vi "def.hReadChannels-UandP-2013.vi"(0 "FPGA VI Reference In":refnum<k20>, 1 "SavGol side points":i32=10, 3 "Use Voltage or Power for AO?":bool, 4 "order polynomial":i32=2, 5 "Nsamples":u32=10000, 6 "error in":errorcluster, 8 "output cluster":T3, 9 "No. Of Samples to average":i32=10, 10 "variables cluster":T2, 11 "calculation settings":i32(slide) scale=0.0..3.0) -> (2 "Fehler":bool, 13 "AdjustedArray":sgl[][](array[numeric]), 18 "single channel voltage array":dbl[](array[numeric]), 19 "real time P_rad array":dbl[](array[numeric]), 20 "FPGA VI Reference Out":refnum<k20>, 22 "PowerArray":sgl[][](array[numeric]), 25 "RawArray":sgl[][](array[numeric]), 26 "error out":errorcluster)   [LabVIEW 2014]
doc: "startet das einlesen und führt dies bis n Samples aus\nHier mit FIFO und IRQ."
uses:
  <vilib>/Utility/error.llb/Error Cluster From Error Code.vi
  <vilib>/rvi/errors/niLvFpgaAdjustHostInterfaceError.vi
  <vilib>/RVI Host/nirviSupport.llb/nirviErrorClusterFromErrorCode.vi
  <vilib>/rvi/interface/nirviReadWriteControl/nirviReadWriteControl.xnode
  FPGA Bitfiles/W7XBolo2017_FPGATarget_fmain2014_DACRangeVoltage.lvbitx
  f_main_2014.vi
  <vilib>/rvi/interface/nirviMethod/nirviMethod.xnode
  NiFpgaLv.dll
  <vilib>/rvi/interface/nirviMethod/StockFPGA_InlinedMethodWaitForMultipleIRQ.vi
  <vilib>/FPGAPlugInAG/PCI-7813R/niLvFpga_WaitOnIrq_PCI-7813R.vi
  <vilib>/FPGAPlugInAG/PCI-7813R/niLvFpga_AcknowledgeIrq_PCI-7813R.vi
  <vilib>/FPGAPlugInAG/PCI-7813R/niLvFpga_ReadFifo_PCI-7813R.vi
  <vilib>/rvi/errors/niLvFpgaMergeErrorWithErrorCode.vi
panel:
  out "current P_rad [MW]":dbl
  out "current power":dbl[](array[numeric])
  out "single channel voltage * factor":dbl
  out "single channel voltage":dbl
  out "dU/dt":sgl[](array[numeric])
  out "channel number":i64
  in  "Tab Control":T1(tab)
  out "16bit integer voltage sample":i16[](array[numeric])=[-3459, -13133, -14604, -16468, 467, -1949, 12299, 12787, 12472, -19409, -24159, 19527, -14453, 13215, 13480, -17931, -19879, 19455, -20502, -24677, -3, 20022, 11523, 10117, 14450, -11995, -12638, 11593, -19028, 12318, 19839, -23479, 32767, -21197, -15773, 20123, 21626, -27672, 23062, -27030, 4395, 3490, 7778, -9544, 25980, -26635, -25599, 29504, 12544, -15434, 16294, -20022, -6530, 14029, -13674, -17269, -19063, -18202, -13922, 21944, -6026, -8393, -17071, -20550, 12209, -14874, -15412, 11029, -20655, 14995, 22414, -12873, 5782, -26944, -17259, 19698, -13837, 22149, 14480, -14147, -12057, 17536, 17816, -16154, -28940, -27971, -27523, -32768, -7372, 9053, 14111, -11921, 20354, -19665, -19289, 15438, -21905, 20094, 19557, -3, 18164, -14518, -19835, 24079, 10990, -13629, -14209, 12810, 4988, -72, 5308, -15, -12833, -7, -34, -7, -7, -11, -62, -4, -6, -7, -47, -5, -8, -29, -17, -1]
  out "RTPRad voltage factor":dbl
  out "Timed Out":bool
  out "STOP?":bool
  out "Elements Remaining":u32
  out "empty sample array":dbl[](array[numeric])
  out "Nsamples array":i64[](array[numeric])
  out "sample":i32
  out "new level of override":i32
  out "last U sample":sgl[](array[numeric])
  out "rt prad average array":dbl[][](array[numeric])
  out "element of channel\nand sample":sgl
  in  "magic number":dbl=1.0
  out "prad av array":dbl[](array[numeric])
  out "RawScal":dbl[](array[numeric])
  out "Scale(mV)":sgl[](array[numeric])
  out "SumScal":dbl[](array[numeric])
  out "Tau/dt":dbl[](array[numeric])
  out "F_ch":dbl[](array[numeric])
  out "tau_fact":dbl[](array[numeric])
  out "kbolott_and_volume":dbl[][](array[numeric])
  out "samples to exclude":u32
  out "single channel number":i64
  out "channelNumber":i32
  out "channelSelection":i64[][](array[numeric])
  out "tau_M":dbl[](array[numeric])
  out "Offsets":dbl[](array[numeric])
  out "SampleTime":sgl
  out "voltage factor":dbl
  out "Scale(mV) transf.":sgl[](array[numeric])
  out "V_cam":dbl
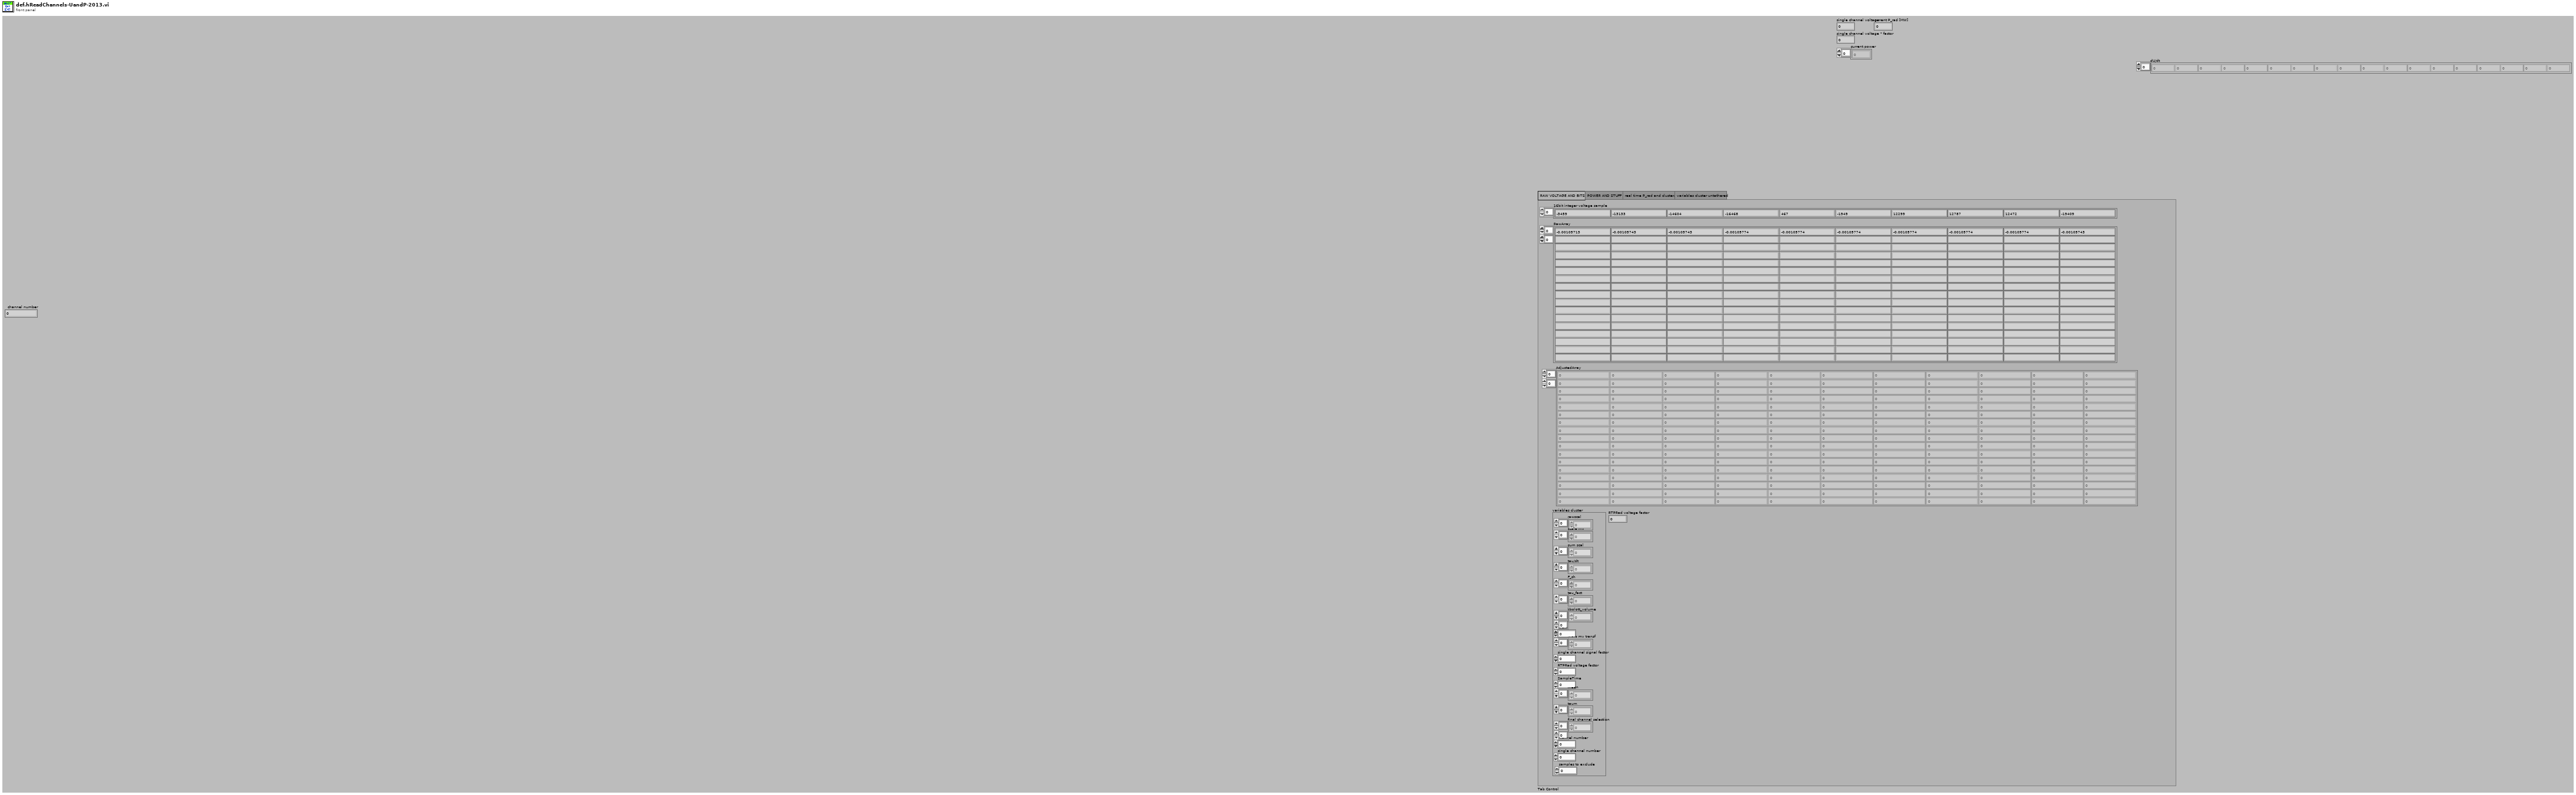
[diagram p1: front panel]
types:
  T1 = enum32{"RAW VOLTAGE AND BITS", "POWER AND STUFF", "real time P_rad and clusters", "variables cluster untathered"}
  T2 = cluster{"rawscal":dbl[], "scale mv":sgl[], "sum scal":dbl[], "tau/dt":dbl[], "F_ch":dbl[], "tau_fact":dbl[], "kbolott_volume":dbl[][], "Vcam":dbl, "scale mv transf":sgl[], "single channel signal factor":dbl, "RTPRad voltage factor":dbl, "SampleTime":sgl, "mean":dbl[], "taum":dbl[], "final channel selection":i64[][], "channel number":i32, "single channel number":i64, "samples to exclude":u32}
  T3 = cluster{"real time P_rad":refnum<vi>, "real time P_rad array":refnum<vi>, "single channel voltage":refnum<vi>, "single channel voltage array":refnum<vi>}
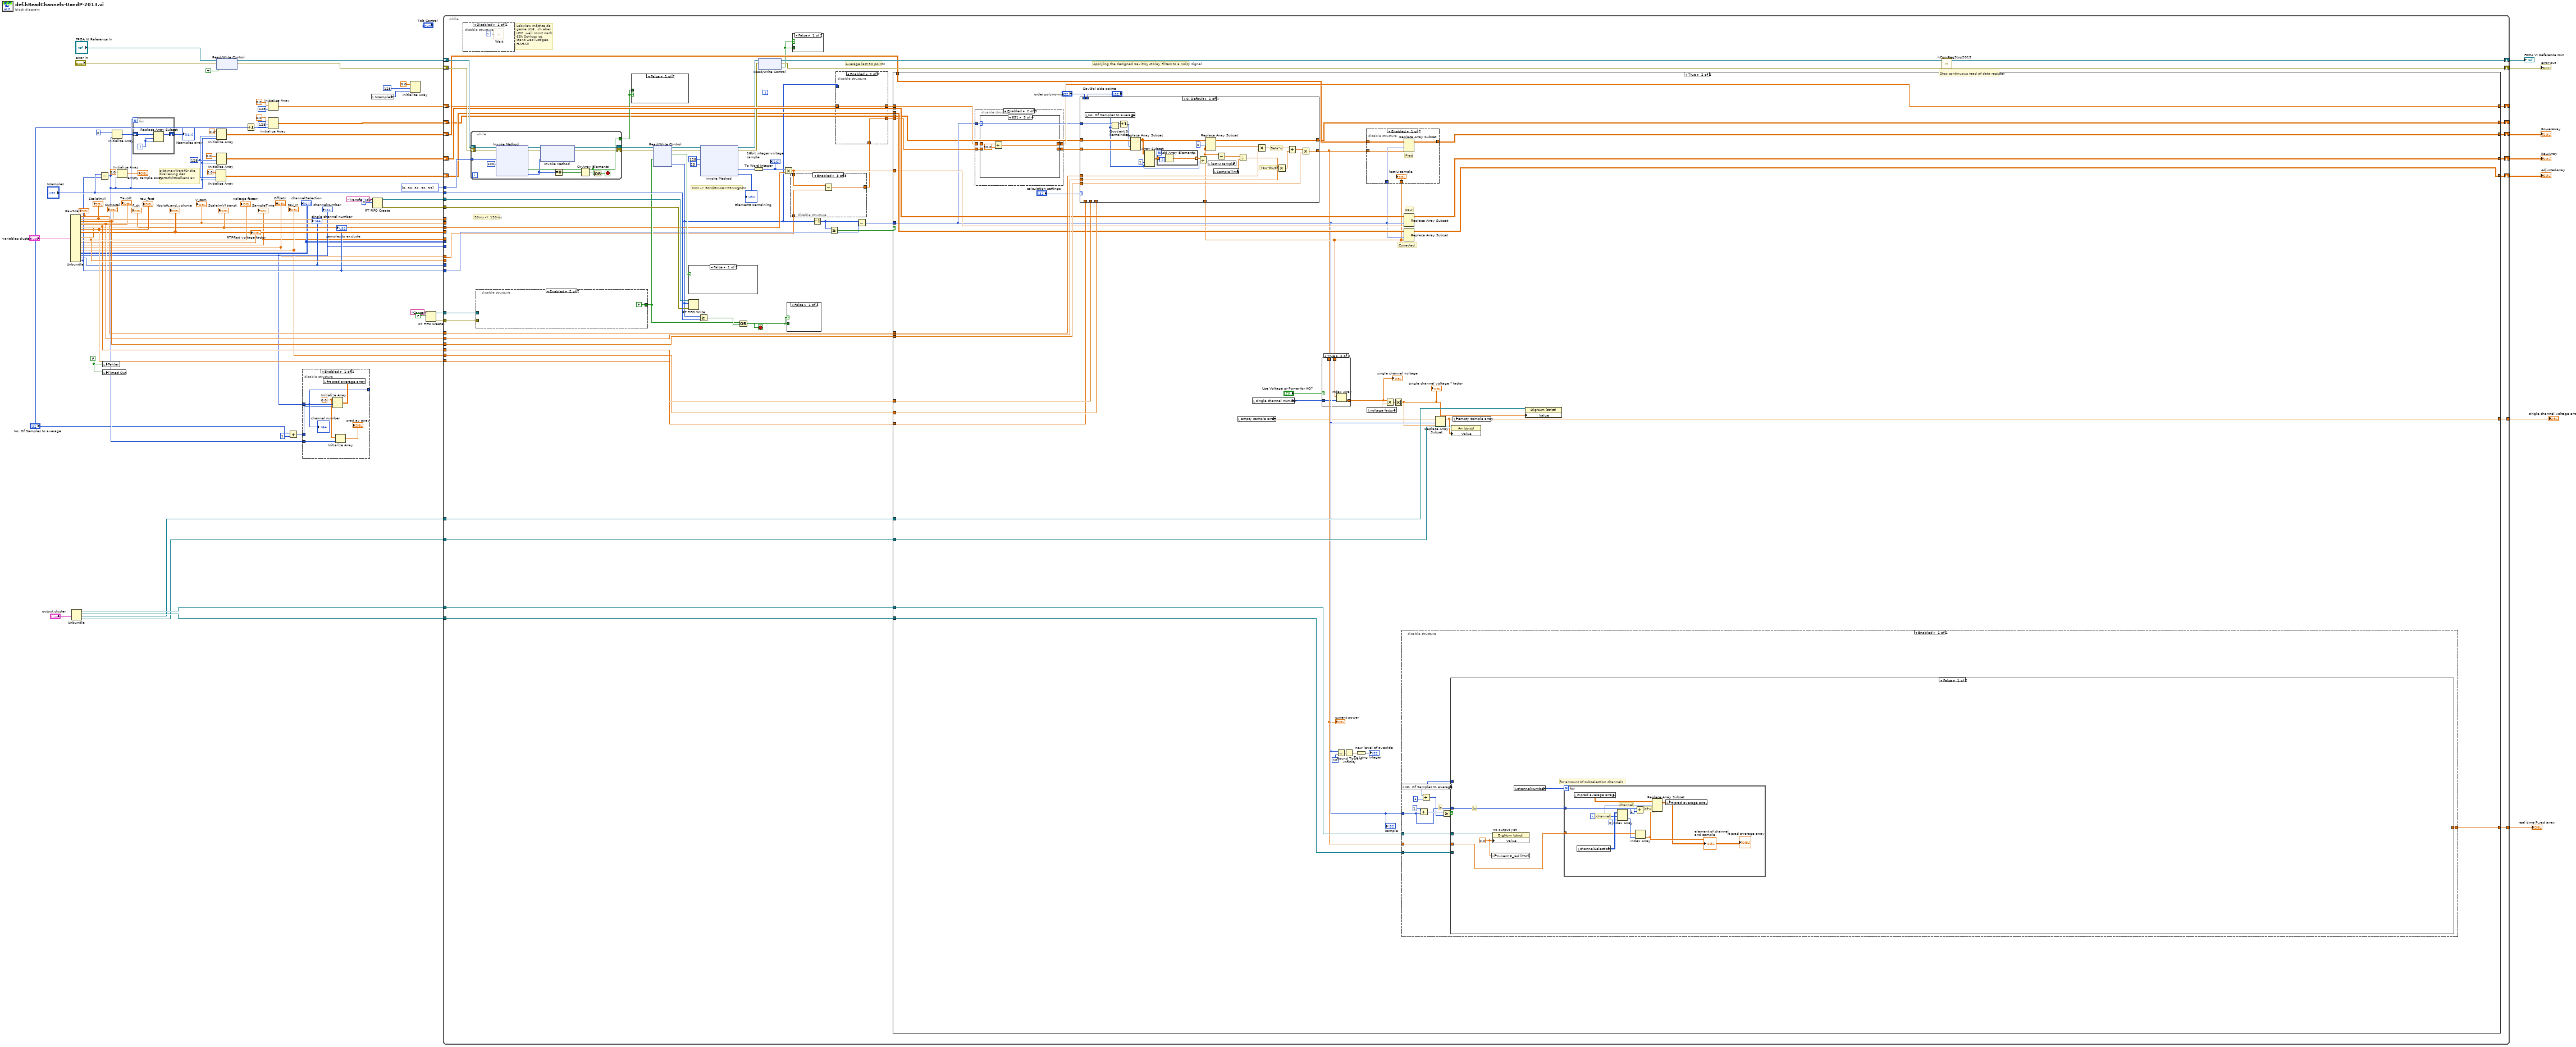
[diagram p0: block diagram]
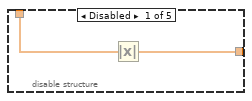
[diagram p2: hidden frame]
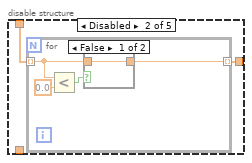
[diagram p3: hidden frame]
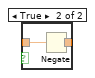
[diagram p4: hidden frame]
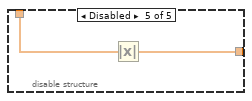
[diagram p6: hidden frame]
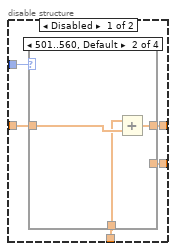
[diagram p7: hidden frame]
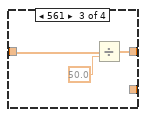
[diagram p9: hidden frame]
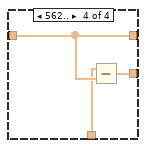
[diagram p10: hidden frame]
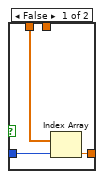
[diagram p12: hidden frame]
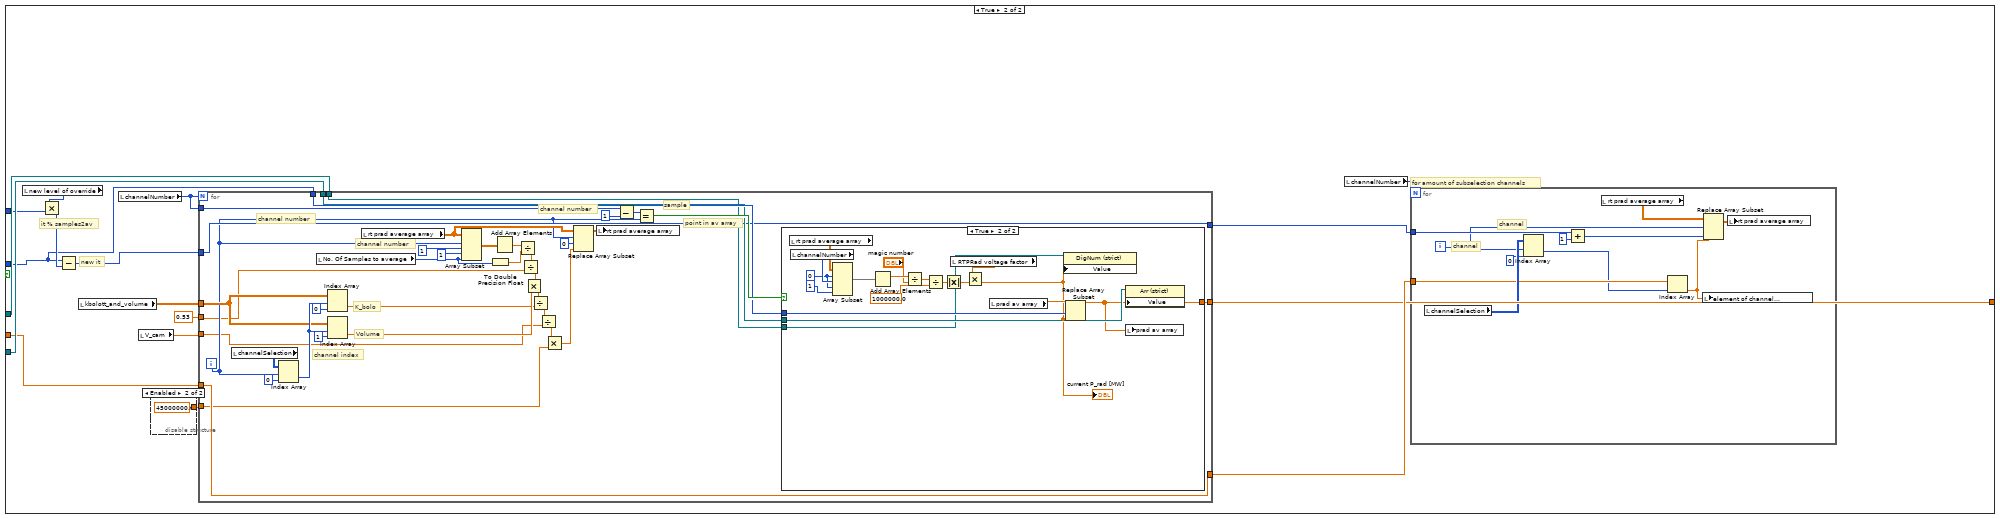
[diagram p13: hidden frame]
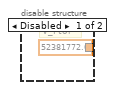
[diagram p14: hidden frame]
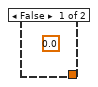
[diagram p15: hidden frame]
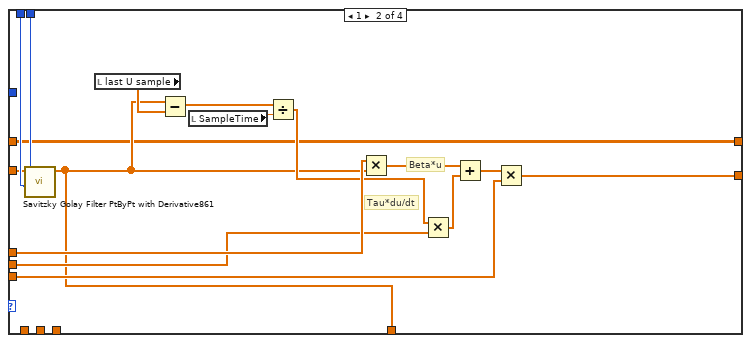
[diagram p17: hidden frame]
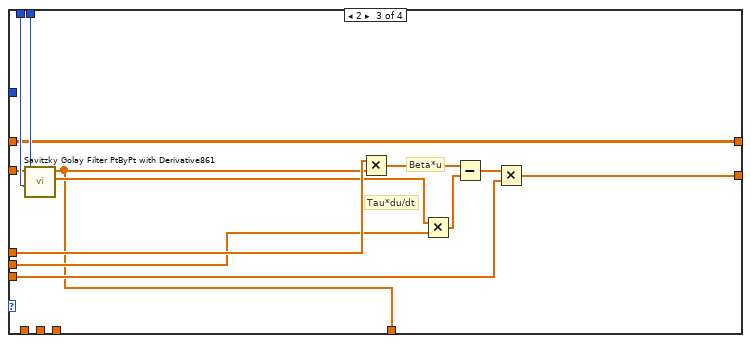
[diagram p18: hidden frame]
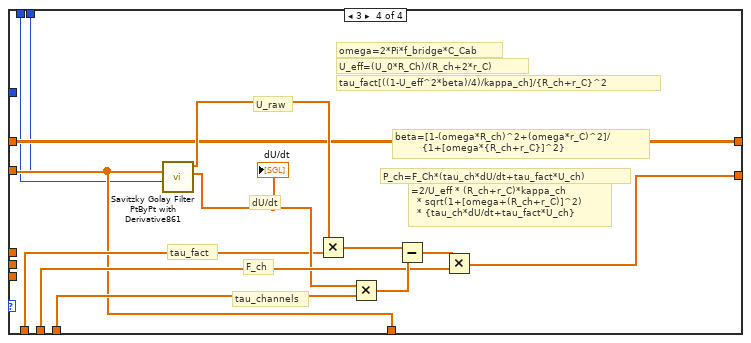
[diagram p19: hidden frame]
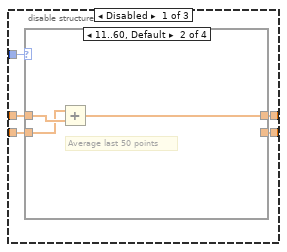
[diagram p20: hidden frame]
diagram:
  w44 = FALSE
  w19 = 128 ("dimension size")
  # "Stop continuous read of data register"
  # "gibt maxWert für die Skalierung des Fortschrittbalkens an"
  n1 = Unbundle("variables cluster") -> ("rawscal"=w35:dbl[], "scale mv"=w30:sgl[], "sum scal"=w36:dbl[], "tau/dt"=w34:dbl[], "F_ch"=w33:dbl[], "tau_fact"=w32:dbl[], "kbolott_volume"=w31:dbl[][], "Vcam"=w28:dbl, "scale mv transf"=w29:sgl[], "single channel signal factor"=w37:dbl, "RTPRad voltage factor"=→"RTPRad voltage factor":dbl, "SampleTime"=w8:sgl, "mean"=w9:dbl[], "taum"=w10:dbl[], "final channel selection"=w11:i64[][], "channel number"=w12:i32, "single channel number"=w13:i64, "samples to exclude"=w14:u32)
  "RawScal" <- w35
  "Scale(mV)" <- w30
  "SumScal" <- w36
  "Tau/dt" <- w34
  "F_ch" <- w33
  "tau_fact" <- w32
  "kbolott_and_volume" <- w31
  "V_cam" <- w28
  "Scale(mV) transf." <- w29
  "voltage factor" <- w37
  "SampleTime" <- w8
  "Offsets" <- w9
  "tau_M" <- w10
  "channelSelection" <- w11
  "channelNumber" <- w12
  "single channel number" <- w13
  "samples to exclude" <- w14
  n2 = Unbundle("output cluster") -> ("real time P_rad"=w39:refnum<vi>, "real time P_rad array"=w38:refnum<vi>, "single channel voltage"=w24:refnum<vi>, "single channel voltage array"=w23:refnum<vi>)
  n3 = Subtract(x="Nsamples", y=w14) -> (x-y=w18:u32)
  n4 = local write "Fehler"(w44) -> ()
  n5 = local write "Timed Out"(w44) -> ()
  n6 = Initialize Array(i64 0 ("element"), w18) -> (w46:i64[])
  n7 = Initialize Array(0.0 ("element"), w18) -> (→"empty sample array":dbl[])
  n8 = for {
    N: w18 -> [_]
    shift-right: [w76] -> w45
    shift-left: w46 -> [w78]
    i -> [w77]
    n9 = Replace Array Subset(array=w78, new element=w77, index=w77) -> (w76:i64[])
  }
  "Nsamples array" <- w45
  n10 = Initialize Array(sgl 0.0 ("element"), w19, w18) -> (w17:sgl[][])
  n11 = xnode "Read/Write Control"("FPGA VI Reference In"="FPGA VI Reference In", "error in"="error in", "ADCRead"=TRUE) -> ("FPGA VI Reference Out"=w57:refnum<k20>, "error out"=w56:errorcluster)
  n12 = Initialize Array(sgl 0.0 ("i"), w19, w18) -> (w66:sgl[][])
  n13 = Initialize Array(sgl 0.0, w19, w18) -> (w75:sgl[][])
  n14 = Increment(x="No. Of Samples to average") -> (x+1=w1:i32)
  n15 = Initialize Array(sgl 0.0 ("element"), 128 ("dimension size")) -> (w52:sgl[])
  n16 = Initialize Array(sgl 0.0 ("element"), 128 ("dimension size"), w1) -> (w3:sgl[][])
  n17 = Add(x="No. Of Samples to average", y=1) -> (x+y=w26:i32)
  n18 = disable-structure shown="Enabled" {
    disable-tunnel: w12 -> [w83]
    disable-tunnel: [w83] -> _
    disable-tunnel: w26 -> [w79]
    disable-tunnel: w18 -> [w80]
    frame Enabled {
      w82 = 0.0 ("element")
      n19 = Initialize Array(w82, w83, w79) -> (w84:dbl[][])
      n20 = local write "rt prad average array"(w84) -> ()
      n21 = Initialize Array(w82, w80) -> (→"prad av array":dbl[])
      "channel number" <- w83
    }
  }
  n22 = local read "Nsamples"() -> (w41:u32)
  n23 = RT FIFO Create(0:"Transferred1" ("name (unnamed)"), 1:u32 0) -> (8:w72:refnum<k33>, 11:w71:errorcluster)  [unwired: 2 in, 5 out]
  n24 = Initialize Array(sgl 0.0 ("element"), 128 ("dimension size"), w41) -> ()  [unwired: 1 out]
  n25 = RT FIFO Create(0:"Cancel" ("name (unnamed)"), 1:FALSE) -> (8:w69:refnum<k33>, 11:w68:errorcluster)  [unwired: 2 in, 5 out]
  n26 = while {
    tunnel: "Nsamples" -> [w139]
    shift-right: [w108] -> w15
    shift-left: w75 -> [w128]
    shift-right: [w140] -> w65
    shift-left: w57 -> [w143]
    shift-right: [w141] -> w64
    shift-left: w56 -> [w142]
    tunnel: w72 -> [w138]
    tunnel: w71 -> [w137]
    tunnel: w69 -> [w135]
    tunnel: w68 -> [w134]
    shift-right: [w132] -> w60
    shift-left: w66 -> [w133]
    tunnel: w29 -> [w127]
    tunnel: w34 -> [w87]
    tunnel: w36 -> [w126]
    tunnel: w35 -> [w125]
    shift-right: [w118] -> _
    shift-left: w52 -> [w94]
    tunnel: i32[] [0, 30, 31, 32, 33] -> [w113]
    tunnel: w23 -> [w110]
    tunnel: w24 -> [w109]
    tunnel: w13 -> [_]
    tunnel: w37 -> [_]
    tunnel: w9 -> [w88]
    tunnel: w14 -> [w89]
    tunnel: w39 -> [w105]
    tunnel: w38 -> [w100]
    tunnel: w33 -> [w104]
    tunnel: w32 -> [w103]
    tunnel: w30 -> [_]
    tunnel: w31 -> [_]
    tunnel: w8 -> [_]
    tunnel: w10 -> [w102]
    tunnel: w11 -> [_]
    tunnel: w12 -> [_]
    tunnel: w28 -> [_]
    tunnel: [w99] -> w22
    tunnel: [w98] -> w21
    shift-right: [w96] -> w16
    shift-left: w17 -> [w97]
    shift-right: [w85] -> _
    shift-left: w3 -> [w86]
    stop <- w114 stop-if-true
    # "Average last 50 points"
    # "Applying the designed Savitzky-Golay Filters to a noisy signal"
    # "LabView möchte da gerne U16, ich aber U32, weil sonst nach 65k Schluss ist. \nGanz was lustiges, HAHA!!"
    # "5ms=>25ms@MM"
    # "0ms -> 50ms"
    # "50ms -> 150ms"
    n27 = disable-structure shown="Disabled" {
      frame Disabled {
        n28 = call "Wait"("Count(uSec)"=u32 5) -> ()  [unwired: 1 out]
      }
      frame Enabled {
      }
    }
    n29 = while {
      tunnel: [w464] -> w117
      shift-right: [w466] -> w111
      shift-left: w143 -> [w473]
      shift-right: [w465] -> w112
      shift-left: w142 -> [w472]
      tunnel: w113 -> [w470]
      stop <- w463 stop-if-true
      n30 = xnode "Invoke Method"("FPGA VI Reference In"=w473, "error in"=w472, "IRQ Number(s)"=w470, "Timeout (ms)"=100) -> ("FPGA VI Reference Out"=w467:refnum<k20>, "error out"=w468:errorcluster, "Timed Out"=w464:bool, "IRQ(s) Asserted"=w469:i32[])
      n31 = xnode "Invoke Method"("FPGA VI Reference In"=w467, "error in"=w468, "IRQ Number(s)"=w469) -> ("FPGA VI Reference Out"=w466:refnum<k20>, "error out"=w465:errorcluster)
      n32 = Equal To 0?(x=w469) -> (x = 0?=w462:bool[])
      n33 = Or Array Elements(Boolean array=w462) -> (logical OR=w461:bool)
      n34 = Or(x=w461, y=w464) -> (x .or. y?=w463:bool)
    }
    n35 = disable-structure shown="Enabled" {
      disable-tunnel: [w479 FALSE] -> w136
      disable-tunnel: w135 -> [w478 _]
      disable-tunnel: w134 -> [w477 _]
      frame Disabled {
        # "Da es passieren kann, dass der letzte IRQ verschluckt wird, sichert dies der Timeoutwert von 50ms ab."
        n36 = RT FIFO Read(0:w478, 1:FALSE ("element"), 3:w477) -> (9:w479:bool)  [unwired: 5 out]
      }
      frame Enabled {
      }
    }
    n37 = case shown="False" w117 {
      tunnel: w117 -> [_ w481]
      frame False {
      }
      frame True {
        "Timed Out" <- w481
      }
    }
    n38 = xnode "Read/Write Control"("FPGA VI Reference In"=w111, "error in"=w112, "cancel"=w136) -> ("FPGA VI Reference Out"=w130:refnum<k20>, "error out"=w129:errorcluster, "Timeout"=w131:bool, "ScanID"=w95:u32)
    n39 = case shown="False" w131 {
      selector: w131 -> [_ w483]
      frame False {
      }
      frame True {
        n40 = local write "Fehler"(w483) -> ()
      }
    }
    n41 = RT FIFO Write(0:w138, 1:w95, 3:w137) -> ()  [unwired: 1 in, 5 out]
    n42 = Greater Or Equal?(x=w95, y=w139) -> (x >= y?=w144:bool)
    n43 = xnode ("Invoke Method")("FPGA VI Reference In"=w130, "error in"=w129, "Number of Elements"=u32 128, "Timeout (ms)"=25 ("Timeout")) -> ("FPGA VI Reference Out"=w120:refnum<k20>, "error out"=w119:errorcluster, "Data"=w122:u32[], "Elements Remaining"=→"Elements Remaining":u32)
    n44 = Compound Arithmetic op=OR(w136, w144) -> (w114:bool)
    n45 = To Word Integer(number=w122) -> (16bit integer=w121:i16[])
    "16bit integer voltage sample" <- w121
    n46 = xnode "Read/Write Control"("FPGA VI Reference In"=w120, "error in"=w119) -> ("FPGA VI Reference Out"=w140:refnum<k20>, "error out"=w141:errorcluster, "Fifo-Fehler"=w115:bool)
    n47 = Multiply(x=w121, y=w127) -> (x*y=w92:sgl[])
    n48 = case shown="False" w114 {
      tunnel: w114 -> [_ w474]
      frame False {
      }
      frame True {
        "STOP?" <- w474
      }
    }
    n49 = disable-structure shown="Enabled" {
      disable-tunnel: [w146 w147 w158 w159 w161] -> w91
      disable-tunnel: w92 -> [w145 w148 w157 w159 w160]
      disable-tunnel: w88 -> [_ _ w156 _ _]
      frame Disabled {
        n50 = Absolute Value(x=w145) -> (abs(x)=w146:sgl[])
      }
      frame Disabled {
        n51 = for {
          tunnel: w148 -> [w150] mode=indexing
          tunnel: [w149] -> w147 mode=indexing
          n52 = Less?(x=w150, y=sgl 0.0) -> (x < y?=w151:bool)
          n53 = case shown="False" w151 {
            tunnel: w150 -> [w153 w155]
            tunnel: [w153 w154] -> w149
            frame False {
            }
            frame True {
              n54 = Negate(x=w155) -> (-x=w154:sgl)
            }
          }
        }
      }
      frame Enabled {
        n55 = Subtract(x=w157, y=w156) -> (x-y=w158:dbl[])
      }
      frame Disabled {
      }
      frame Disabled {
        n56 = Absolute Value(x=w160) -> (abs(x)=w161:sgl[])
      }
    }
    n57 = case shown="False" w115 {
      tunnel: w115 -> [_ w475]
      frame False {
      }
      frame True {
        "Fehler" <- w475
      }
    }
    n58 = Decrement(x=w95) -> (x-1=w106:u32)
    n59 = Greater Or Equal?(x=w106, y=w89) -> (x >= y?=w107:bool)
    n60 = disable-structure shown="Enabled" {
      disable-tunnel: [w166 w178] -> w93
      disable-tunnel: w94 -> [w165 w178]
      disable-tunnel: w95 -> [w164 _]
      disable-tunnel: [w163 w177] -> w90
      disable-tunnel: w91 -> [w162 w177]
      frame Disabled {
        n61 = case shown="501..560, Default" w164 {
          tunnel: w162 -> [_ w168 _ w174]
          tunnel: [w167 w170 w171 w175] -> w166
          tunnel: w165 -> [w167 w169 w173 w175]
          tunnel: [_ _ _ w176] -> w163
          frame 0..500 {
          }
          frame 501..560, Default {
            n62 = Add(x=w168, y=w169) -> (x+y=w170:dbl[])
          }
          frame 561 {
            n63 = Divide(x=w173, y=sgl 50.0) -> (x/y=w171:dbl[])
          }
          frame 562.. {
            n64 = Subtract(x=w174, y=w175) -> (x-y=w176:dbl[])
          }
        }
      }
      frame Enabled {
      }
    }
    n65 = Subtract(x=w106, y=w89) -> (x-y=w101:u32)
    n66 = case shown="True" w107 {
      tunnel: w133 -> [w182 w218]
      tunnel: [w182 w219] -> w132
      tunnel: w128 -> [w181 w217]
      tunnel: w126 -> [_ w225]
      tunnel: w125 -> [_ w224]
      tunnel: w87 -> [_ w223]
      tunnel: [w183 w222] -> w118
      tunnel: w93 -> [w183 w206]
      tunnel: w92 -> [_ w205]
      tunnel: w110 -> [_ w221]
      tunnel: w109 -> [_ w220]
      tunnel: [w181 w216] -> w108
      tunnel: w101 -> [_ w203]
      tunnel: w105 -> [_ w212]
      tunnel: w100 -> [_ w211]
      tunnel: w104 -> [_ w215]
      tunnel: w103 -> [_ w213]
      tunnel: w102 -> [_ w214]
      tunnel: [_ w210] -> w99
      tunnel: [_ w209] -> w98
      tunnel: w97 -> [w180 w208]
      tunnel: [w180 w207] -> w96
      tunnel: w90 -> [_ w204]
      tunnel: w86 -> [w179 w202]
      tunnel: [w179 w201] -> w85
      frame False {
      }
      frame True {
        # "Corrected"
        # "Raw"
        n67 = disable-structure shown="Enabled" {
          disable-tunnel: [w416 w442 w453] -> w222
          disable-tunnel: w206 -> [w415 w441 w453]
          disable-tunnel: w203 -> [w414 w440 _]
          disable-tunnel: [w413 w439 w454] -> w196
          disable-tunnel: w204 -> [w412 w438 w454]
          frame Disabled {
            n68 = case shown="11..60, Default" w414 {
              tunnel: w412 -> [_ w418 _ w434]
              tunnel: [w417 w420 w422 w433] -> w416
              tunnel: w415 -> [w417 w419 w424 w433]
              tunnel: [_ _ _ w432] -> w413
              frame 0..10 {
              }
              frame 11..60, Default {
                # "Average last 50 points"
                n69 = Add(x=w418, y=w419) -> (x+y=w420:dbl[])
              }
              frame 61 {
                n70 = Divide(x=w424, y=sgl 50.0) -> (x/y=w421:dbl[])
                n71 = disable-structure shown="Enabled" {
                  disable-tunnel: [w425 w430] -> w422
                  disable-tunnel: w421 -> [w429 w430]
                  frame Disabled {
                    n72 = Initialize Array(2e-06 ("element"), 128 ("dimension size")) -> (w426:dbl[])
                    n73 = Subtract(x=w429, y=w426) -> (x-y=w425:dbl[])
                  }
                  frame Enabled {
                  }
                }
              }
              frame 62.. {
                n74 = Subtract(x=w434, y=w433) -> (x-y=w431:dbl[])
                n75 = disable-structure shown="Enabled" {
                  disable-tunnel: [w436 w437] -> w432
                  disable-tunnel: w431 -> [w435 w437]
                  frame Disabled {
                    n76 = Absolute Value(x=w435) -> (abs(x)=w436:dbl[])
                  }
                  frame Enabled {
                  }
                }
              }
            }
          }
          frame Enabled {
            n77 = case shown="651" w440 {
              tunnel: w438 -> [_ w444 _ w452]
              tunnel: [w443 w446 w447 w451] -> w442
              tunnel: w441 -> [w443 w445 w449 w451]
              tunnel: [_ _ _ w450] -> w439
              frame 0..600 {
              }
              frame 601..650, Default {
                # "Average last 50 points"
                n78 = Add(x=w444, y=w445) -> (x+y=w446:dbl[])
              }
              frame 651 {
                n79 = Divide(x=w449, y=sgl 50.0) -> (x/y=w447:dbl[])
              }
              frame 652.. {
                n80 = Subtract(x=w452, y=w451) -> (x-y=w450:dbl[])
              }
            }
          }
          frame Disabled {
          }
        }
        n81 = case shown="0, Default" "calculation settings" {
          tunnel: w225 -> [w367 w385 w398 _]
          tunnel: w224 -> [w366 w384 w397 _]
          tunnel: w223 -> [w365 w383 w396 _]
          tunnel: [w364 w382 w395 w403] -> w199
          tunnel: "SavGol side points" -> [_ w381 w394 w400]
          tunnel: "order polynomial" -> [_ w380 w393 w399]
          tunnel: w196 -> [w363 w379 w392 w401]
          tunnel: w203 -> [w362 _ _ _]
          tunnel: w202 -> [w361 w370 w387 w402]
          tunnel: [w360 w370 w387 w402] -> w201
          tunnel: [w359 w371 w386 w401] -> w200
          tunnel: w214 -> [_ _ _ w407]
          tunnel: w215 -> [_ _ _ w406]
          tunnel: w213 -> [_ _ _ w404]
          frame 0, Default {
            # "Beta*u"
            # "Tau*du/dt"
            n82 = local read "No. Of Samples to average"() -> (w353:i32)
            n83 = Quotient & Remainder(x=w362, y=w353) -> (x-y*floor(x/y)=w357:u32)  [unwired: 1 out]
            n84 = Increment(x=w357) -> (x+1=w358:u32)
            n85 = Replace Array Subset(array=w361, new element=w363, index (col)=w358) -> (w352:sgl[][])  [unwired: 1 in]
            n86 = Array Subset(array=w352, index (col)=1 ("index"), length (col)=w353) -> (w355:sgl[][])  [unwired: 2 in]
            n87 = for {
              tunnel: w355 -> [w369] mode=indexing
              tunnel: [w368] -> w354 mode=indexing
              n88 = Add Array Elements(numeric array=w369) -> (sum=w368:sgl)
            }
            n89 = Divide(x=w354, y=w353) -> (x/y=w359:sgl[])
            n90 = Replace Array Subset(array=w352, new element=w359, index (col)=0 ("index")) -> (w360:sgl[][])  [unwired: 1 in]
            n91 = local read "last U sample"() -> (w350:sgl[])
            n92 = local read "SampleTime"() -> (w348:sgl)
            n93 = Subtract(x=w359, y=w350) -> (x-y=w349:sgl[])
            n94 = Divide(x=w349, y=w348) -> (x/y=w344:sgl[])
            n95 = Multiply(x=w359, y=w366) -> (x*y=w347:dbl[])
            n96 = Multiply(x=w344, y=w365) -> (x*y=w345:dbl[])
            n97 = Add(x=w347, y=w345) -> (x+y=w346:dbl[])
            n98 = Multiply(x=w346, y=w367) -> (x*y=w364:dbl[])
          }
          frame 1 {
            # "Beta*u"
            # "Tau*du/dt"
            n99 = call "Savitzky Golay Filter PtByPt with Derivative861.vi"("order polynomial"=w380, "side points"=w381, "x"=w379) -> ("Filtered x"=w371:dbl[])  [unwired: 1 in, 7 out]
            n100 = local read "last U sample"() -> (w373:sgl[])
            n101 = Subtract(x=w371, y=w373) -> (x-y=w374:dbl[])
            n102 = local read "SampleTime"() -> (w372:sgl)
            n103 = Divide(x=w374, y=w372) -> (x/y=w376:dbl[])
            n104 = Multiply(x=w384, y=w371) -> (x*y=w378:dbl[])
            n105 = Multiply(x=w376, y=w383) -> (x*y=w375:dbl[])
            n106 = Add(x=w378, y=w375) -> (x+y=w377:dbl[])
            n107 = Multiply(x=w377, y=w385) -> (x*y=w382:dbl[])
          }
          frame 2 {
            # "Beta*u"
            # "Tau*du/dt"
            n108 = call "Savitzky Golay Filter PtByPt with Derivative861.vi"("order polynomial"=w393, "side points"=w394, "x"=w392) -> ("Filtered Derivative"=w388:dbl[], "Filtered x"=w386:dbl[])  [unwired: 1 in, 6 out]
            n109 = Multiply(x=w397, y=w386) -> (x*y=w391:dbl[])
            n110 = Multiply(x=w388, y=w396) -> (x*y=w389:dbl[])
            n111 = Subtract(x=w391, y=w389) -> (x-y=w390:dbl[])
            n112 = Multiply(x=w390, y=w398) -> (x*y=w395:dbl[])
          }
          frame 3 {
            # "beta=[1-(omega*R_ch)^2+(omega*r_C)^2]/\n         {1+[omega*{R_ch+r_C}]^2}"
            # "tau_fact[((1-U_eff^2*beta)/4)/kappa_ch]/{R_ch+r_C}^2"
            # "U_eff=(U_0*R_Ch)/(R_ch+2*r_C)"
            # "omega=2*Pi*f_bridge*C_Cab"
            # "=2/U_eff * (R_ch+r_C)*kappa_ch\n  * sqrt(1+[omega+(R_ch+r_C)]^2)\n  * {tau_ch*dU/dt+tau_fact*U_ch}"
            # "P_ch=F_Ch*(tau_ch*dU/dt+tau_fact*U_ch)"
            # "tau_channels"
            # "F_ch"
            # "tau_fact"
            # "U_raw"
            # "dU/dt"
            n113 = call "Savitzky Golay Filter PtByPt with Derivative861.vi"("order polynomial"=w399, "side points"=w400, "x"=w401) -> ("Filtered Derivative"=w405:dbl[], "Filtered x"=w408:dbl[])  [unwired: 1 in, 6 out]
            "dU/dt" <- w405
            n114 = Multiply(x=w408, y=w404) -> (x*y=w411:dbl[])
            n115 = Multiply(x=w405, y=w407) -> (x*y=w409:dbl[])
            n116 = Subtract(x=w411, y=w409) -> (x-y=w410:dbl[])
            n117 = Multiply(x=w410, y=w406) -> (x*y=w403:dbl[])
          }
        }
        "current power" <- w199
        n118 = local read "empty sample array"() -> (w192:dbl[])
        n119 = local read "single channel number"() -> (w194:i64)
        n120 = case shown="True" "Use Voltage or Power for AO?" {
          tunnel: w194 -> [w226 w231]
          tunnel: [w227 w230] -> w191
          tunnel: w200 -> [_ w229]
          tunnel: w199 -> [w228 _]
          frame False {
            n121 = Index Array(array=w228, index=w226) -> (element=w227:dbl)
          }
          frame True {
            n122 = Index Array(array=w229, index=w231) -> (element=w230:dbl)
          }
        }
        "single channel voltage" <- w191
        n123 = Divide(x=w203, y=10) -> (x/y=w187:dbl)
        n124 = Round Toward -Infinity(1:w187) -> (0:w188:dbl)
        n125 = To Long Integer(number=w188) -> (32bit integer=→"new level of override":i32)
        n126 = disable-structure shown="Enabled" {
          disable-tunnel: w218 -> [w459 w460]
          disable-tunnel: [w458 w460] -> w219
          disable-tunnel: w203 -> [w457 _]
          disable-tunnel: w199 -> [w456 _]
          disable-tunnel: w200 -> [w455 _]
          frame Enabled {
            # "Prad"
            n127 = Replace Array Subset(array=w459, new element=w456, index (col)=w457) -> (w458:sgl[][])  [unwired: 1 in]
            "last U sample" <- w455
          }
          frame Disabled {
          }
        }
        n128 = local read "voltage factor"() -> (w193:dbl)
        n129 = Multiply(x=w191, y=w193) -> (x*y=w190:dbl)
        n130 = Absolute Value(x=w190) -> (abs(x)=w184:dbl)
        "single channel voltage * factor" <- w184
        n131 = disable-structure shown="Enabled" {
          disable-tunnel: w203 -> [w236 _]
          disable-tunnel: w212 -> [w239 _]
          disable-tunnel: w211 -> [w238 _]
          disable-tunnel: w199 -> [w237 _]
          disable-tunnel: [w232 _] -> w210
          frame Enabled {
            # "it"
            n132 = local read "No. Of Samples to average"() -> (w233:i32)
            n133 = Add(x=1, y=w236) -> (x+y=w240:u32)
            n134 = Add(x=w233, y=i64 1) -> (x+y=w234:i64)
            n135 = Greater Or Equal?(x=w240, y=w234) -> (x >= y?=w242:bool)
            n136 = case shown="False" w242 {
              tunnel: w236 -> [w244 w261]
              tunnel: w239 -> [w246 w263]
              tunnel: w238 -> [_ w264]
              tunnel: w237 -> [w245 w262]
              tunnel: w233 -> [_ w260]
              tunnel: [_ w259] -> w232
              frame False {
                w243 = 0.0 ("Value")
                # "it"
                # "for amount of subselection channels"
                # "no output yet"
                n137 = local write "current P_rad [MW]"(w243) -> ()
                n138 = property class="DigNum (strict)"(reference=w246, "Value"=w243) -> ()  [unwired: 1 in, 2 out]
                n139 = local read "channelNumber"() -> (w247:i32)
                n140 = for {
                  N: w247 -> [_]
                  tunnel: w244 -> [w254]
                  tunnel: w245 -> [w252]
                  i -> [w249]
                  # "channel"
                  # "channel"
                  # "it+1"
                  n141 = local read "rt prad average array"() -> (w253:dbl[][])
                  n142 = local read "channelSelection"() -> (w258:i64[][])
                  n143 = Index Array(array=w258, index (row)=w249, index (col)=0 ("disabled index (col)")) -> (element=w248:i64)
                  n144 = Add(x=w254, y=1) -> (x+y=w255:u32)
                  n145 = Index Array(array=w252, index=w248) -> (element=w251:dbl)
                  "element of channel\nand sample" <- w251
                  n146 = Replace Array Subset(array=w253, new element=w251, index (row)=w249, index (col)=w255) -> (w250:dbl[][])
                  "rt prad average array" <- w250
                  n147 = local write "rt prad average array"(w250) -> ()
                }
              }
              frame True {
                # "new it"
                # "it % samples2av"
                # "for amount of subselection channels"
                n148 = local read "new level of override"() -> (w274:i32)
                n149 = Multiply(x=w274, y=w260) -> (x*y=w273:i32)
                n150 = Subtract(x=w261, y=w273) -> (x-y=w271:u32)
                n151 = local read "kbolott_and_volume"() -> (w272:dbl[][])
                n152 = local read "channelNumber"() -> (w266:i32)
                n153 = local read "V_cam"() -> (w268:dbl)
                n154 = disable-structure shown="Enabled" {
                  disable-tunnel: [52381772.0 45000000.0] -> w270
                  frame Disabled {
                    # "V_Ptor"
                  }
                  frame Enabled {
                  }
                }
                n155 = for {
                  N: w266 -> [_]
                  tunnel: w272 -> [w309]
                  tunnel: [w314] -> w267
                  tunnel: w262 -> [w314]
                  tunnel: [w294] -> w265
                  tunnel: w271 -> [w294]
                  tunnel: w270 -> [w288]
                  tunnel: 0.53 -> [w292]
                  tunnel: w268 -> [w289]
                  tunnel: w266 -> [w295]
                  tunnel: w261 -> [w300]
                  tunnel: w264 -> [w299]
                  tunnel: w263 -> [w296]
                  tunnel: [w279] -> w259
                  i -> [w293]
                  # "channel number"
                  # "channel number"
                  # "point in av array"
                  # "sample"
                  # "channel number"
                  # "K_bolo"
                  # "Volume"
                  # "channel index"
                  n156 = local read "channelSelection"() -> (w313:i64[][])
                  n157 = Index Array(array=w313, index (row)=w293, index (col)=0 ("disabled index (col)")) -> (element=w310:i64)
                  n158 = local read "No. Of Samples to average"() -> (w281:i32)
                  n159 = Index Array(array=w309, index (row)=w310, index (col)=0 ("disabled index (col)")) -> (element=w290:dbl)
                  n160 = Index Array(array=w309, index (row)=w310, index (col)=1 ("disabled index (col)")) -> (element=w291:dbl)
                  n161 = local read "rt prad average array"() -> (w304:dbl[][])
                  n162 = Array Subset(array=w304, index (row)=w293, length (row)=1, index (col)=1 ("index"), length (col)=w281) -> (w305:dbl[][])
                  n163 = To Double Precision Float(number=w281) -> (double precision float=w280:dbl)
                  n164 = Add Array Elements(numeric array=w305) -> (sum=w286:dbl)
                  n165 = Divide(x=w286, y=w280) -> (x/y=w278:dbl)
                  n166 = Divide(x=w278, y=w292) -> (x/y=w285:dbl)
                  n167 = Multiply(x=w285, y=w291) -> (x*y=w284:dbl)
                  n168 = Divide(x=w284, y=w290) -> (x/y=w283:dbl)
                  n169 = Divide(x=w283, y=w289) -> (x/y=w282:dbl)
                  n170 = Multiply(x=w282, y=w288) -> (x*y=w287:dbl)
                  n171 = Replace Array Subset(array=w304, new element=w287, index (row)=w293, index (col)=0 ("disabled index (col)")) -> (w302:dbl[][])
                  n172 = local write "rt prad average array"(w302) -> ()
                  n173 = Subtract(x=w295, y=i64 1) -> (x-y=w298:i64)
                  n174 = Equal?(x=w298, y=w293) -> (x = y?=w301:bool)
                  n175 = case shown="True" w301 {
                    tunnel: w300 -> [_ w329]
                    tunnel: w299 -> [_ w328]
                    tunnel: w296 -> [_ w327]
                    tunnel: [_ w318] -> w279
                    frame False {
                      (unwired) 0.0
                    }
                    frame True {
                      w324 = 0 ("index")
                      n176 = local read "rt prad average array"() -> (w330:dbl[][])
                      n177 = local read "channelNumber"() -> (w325:i32)
                      n178 = Array Subset(array=w330, index (row)=w324, length (row)=w325, index (col)=w324, length (col)=1 ("index")) -> (w332:dbl[][])
                      n179 = Add Array Elements(numeric array=w332) -> (sum=w322:dbl)
                      n180 = Divide(x=w322, y="magic number") -> (x/y=w323:dbl)
                      n181 = Divide(x=w323, y=1000000.0) -> (x/y=w319:dbl)
                      n182 = Absolute Value(x=w319) -> (abs(x)=w317:dbl)
                      n183 = local read "RTPRad voltage factor"() -> (w316:dbl)
                      n184 = Multiply(x=w316, y=w317) -> (x*y=w315:dbl)
                      "current P_rad [MW]" <- w315
                      n185 = local read "prad av array"() -> (w320:dbl[])
                      n186 = property class="DigNum (strict)"(reference=w327, "Value"=w315) -> ()  [unwired: 1 in, 2 out]
                      n187 = Replace Array Subset(array=w320, new element=w315, index=w329) -> (w318:dbl[])
                      n188 = property class="Arr (strict)"(reference=w328, "Value"=w318) -> ()  [unwired: 1 in, 2 out]
                      n189 = local write "prad av array"(w318) -> ()
                    }
                  }
                }
                n190 = local read "channelNumber"() -> (w275:i32)
                n191 = for {
                  N: w275 -> [_]
                  tunnel: w265 -> [w339]
                  tunnel: w267 -> [w337]
                  i -> [w335]
                  # "channel"
                  # "channel"
                  n192 = local read "channelSelection"() -> (w343:i64[][])
                  n193 = Index Array(array=w343, index (row)=w335, index (col)=0 ("disabled index (col)")) -> (element=w333:i64)
                  n194 = Add(x=w339, y=1) -> (x+y=w340:u32)
                  n195 = local read "rt prad average array"() -> (w338:dbl[][])
                  n196 = Index Array(array=w337, index=w333) -> (element=w334:dbl)
                  n197 = local write "element of channel\nand sample"(w334) -> ()
                  n198 = Replace Array Subset(array=w338, new element=w334, index (row)=w335, index (col)=w340) -> (w336:dbl[][])
                  n199 = local write "rt prad average array"(w336) -> ()
                }
              }
            }
          }
          frame Disabled {
          }
        }
        n200 = Replace Array Subset(array=w217, new element=w205, index (col)=w203) -> (w216:sgl[][])  [unwired: 1 in]
        n201 = Replace Array Subset(array=w208, new element=w200, index (col)=w203) -> (w207:sgl[][])  [unwired: 1 in]
        n202 = Replace Array Subset(array=w192, new element=w184, index=w203) -> (w209:dbl[])
        n203 = property class="Arr (strict)"(reference=w221, "Value"=w209) -> ()  [unwired: 1 in, 2 out]
        n204 = local write "empty sample array"(w209) -> ()
        n205 = property class="DigNum (strict)"(reference=w220, "Value"=w184) -> ()  [unwired: 1 in, 2 out]
        "sample" <- w203
      }
    }
  }
  "RawArray" <- w15
  "PowerArray" <- w60
  "real time P_rad array" <- w22
  "single channel voltage array" <- w21
  "AdjustedArray" <- w16
  n206 = call "hComRegStop2013.vi"("error in"=w64, "FPGA VI Reference In"=w65) -> ("error out"=→"error out":errorcluster, "FPGA VI Reference Out"=→"FPGA VI Reference Out":refnum<k20>)  [unwired: 3 in, 1 out]
